vi "RPC Application.vi"() -> ()   [LabVIEW 2015]
uses:
  Classes/Request/Request.lvclass/Request.ctl
  Classes/Request/Read method.vi
  Classes/Request/Read params.vi
  <vilib>/NI/i3 JSON/JSON Generation/Create Value Files/Create Value - String.vi
  Classes/Server/Add Response (Method Not Found from Request).vi
  <vilib>/NI/i3 JSON/JSON Parsing/Get Array Value at Index Files/Get Array Value at Index - Numeric.vi
  <vilib>/NI/i3 JSON/JSON Generation/Create Value Files/Create Value - Numeric.vi
  Classes/Server/Add Response (Result from Request).vi
  Classes/Server/Add Response (Invalid Params from Request).vi
  Classes/Server/Add Response (Server Error from Request).vi
  Classes/params/params.lvclass
  Classes/Server/JSONRPC Server.lvclass
  <vilib>/NI/i3 JSON/i3-json.lvlib
  Classes/Request/Request.lvclass
panel:
  out "error out":errorcluster
  in  "error in (no error)":errorcluster
  # "To run this example:\n\nStart this VI\nRun \"RPC UI.vi\""
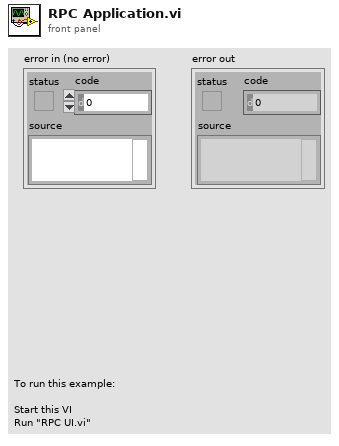
[diagram p1: front panel]
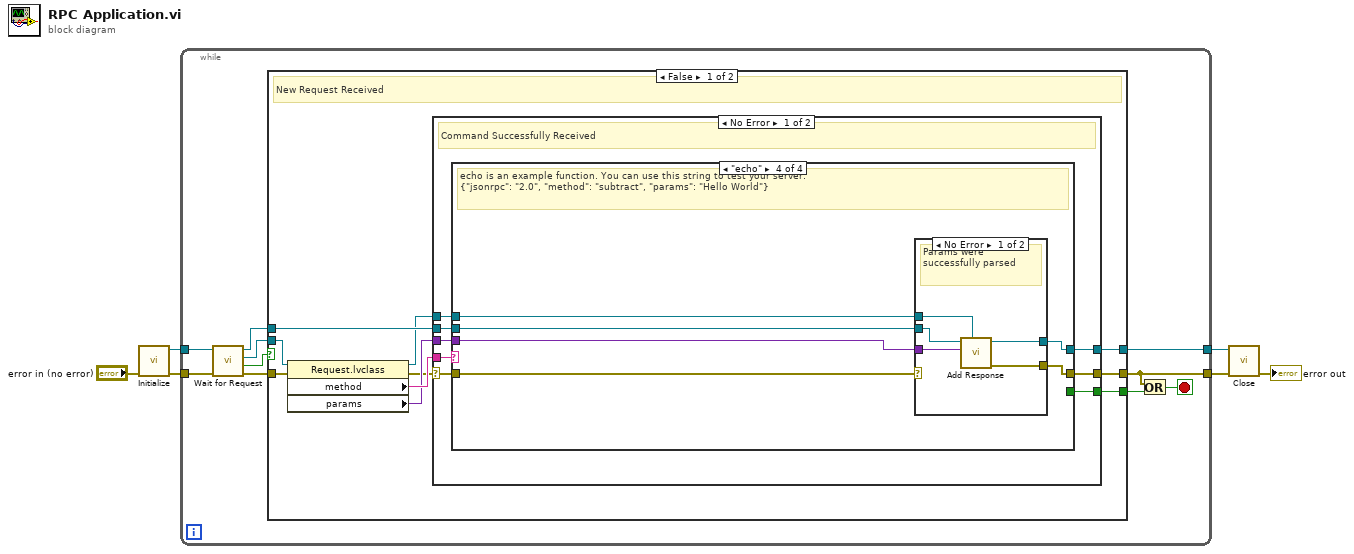
[diagram p0: block diagram]
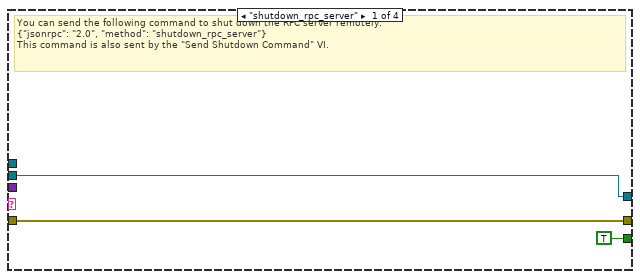
[diagram p2: hidden frame]
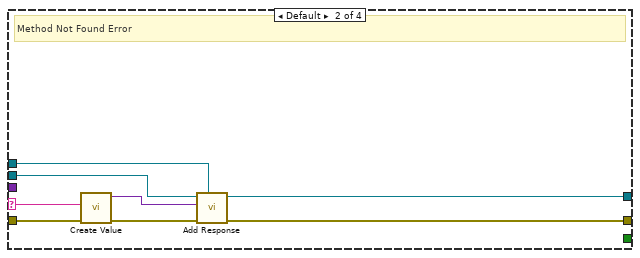
[diagram p3: hidden frame]
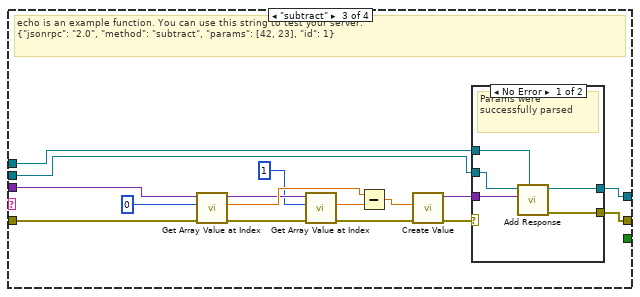
[diagram p4: hidden frame]
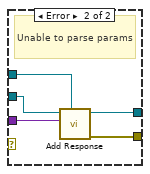
[diagram p5: hidden frame]
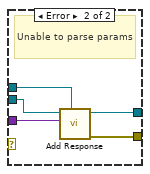
[diagram p6: hidden frame]
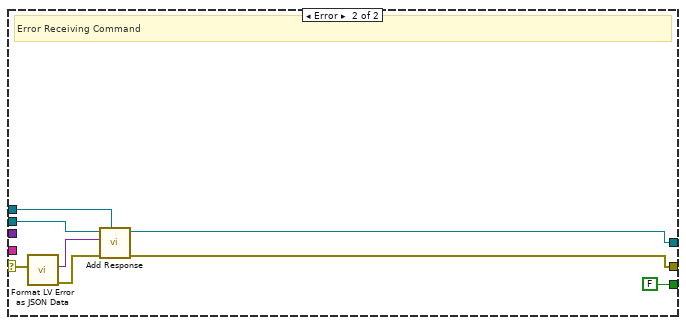
[diagram p7: hidden frame]
diagram:
  n1 = call "Initialize.vi"("error in (no error)"="error in (no error)") -> ("error out"=w2:errorcluster, "Server Out"=w1:refnum<class "JSONRPC Server.lvclass">)  [unwired: 9 in]
  n2 = while {
    tunnel: w1 -> [w16]
    tunnel: w2 -> [w12]
    tunnel: [w8] -> w4
    tunnel: [w10] -> w3
    stop <- w7 stop-if-true
    n3 = call "Wait for Request.vi"("error in (no error)"=w12, "Server in"=w16) -> ("error out"=w11:errorcluster, "timed out?"=w13:bool, "Request"=w14:refnum<class "Request.lvclass">, "Server out"=w15:refnum<class "JSONRPC Server.lvclass">)  [unwired: 6 in]
    n4 = case shown="False" w13 {
      tunnel: w15 -> [w19 w96]
      tunnel: w14 -> [w26 _]
      tunnel: w11 -> [w23 w97]
      tunnel: [w21 w97] -> w8
      tunnel: [w20 _] -> w9
      tunnel: [w18 w96] -> w10
      frame False {
        # "New Request Received"
        n5 = property class="Request.lvclass"(reference=w26, error in=w23) -> (reference out=w17:refnum<class "Request.lvclass">, error out=w22:errorcluster, "method"=w25:string, "params"=w24:variant)
        n6 = case shown="No Error" w22 {
          selector: w22 -> [w32 w89]
          tunnel: w25 -> [w34 _]
          tunnel: w24 -> [w33 _]
          tunnel: [w31 w92] -> w21
          tunnel: [w30 FALSE] -> w20
          tunnel: w19 -> [w29 w94]
          tunnel: [w28 w93] -> w18
          tunnel: w17 -> [w27 w95]
          frame No Error {
            # "Command Successfully Received"
            n7 = case shown="\"echo\"" w34 {
              selector: w34 -> [_ w43 _ _]
              tunnel: w33 -> [_ _ w58 w72]
              tunnel: w32 -> [w36 w39 w56 w73]
              tunnel: [w36 w41 w48 w75] -> w31
              tunnel: [TRUE _ _ _] -> w30
              tunnel: w29 -> [w35 w45 w51 w77]
              tunnel: [w35 w40 w50 w76] -> w28
              tunnel: w27 -> [_ w44 w47 w74]
              frame "shutdown_rpc_server" {
                # "You can send the following command to shut down the RPC server remotely:\n{\"jsonrpc\": \"2.0\", \"method\": \"shutdown_rpc_server\"}\nThis command is also sent by the \"Send Shutdown Command\" VI."
              }
              frame Default {
                # "Method Not Found Error"
                n8 = call-poly <vilib>:"Create Value.vi"("error in (no error)"=w39, "String"=w43) -> ("error out"=w38:errorcluster, "JSON Tree"=w42:variant)  [unwired: 8 in]
                n9 = call-poly "Add Response.vi"("Request"=w44, "error in (no error)"=w38, "data"=w42, "Server in"=w45) -> ("error out"=w41:errorcluster, "Server out"=w40:refnum<class "JSONRPC Server.lvclass">)  [unwired: 6 in]
              }
              frame "subtract" {
                # "echo is an example function. You can use this string to test your server:\n{\"jsonrpc\": \"2.0\", \"method\": \"subtract\", \"params\": [42, 23], \"id\": 1}"
                n10 = call-poly <vilib>:"Get Array Value at Index.vi"("error in (no error)"=w56, "Index"=0, "JSON Tree In (JSON Array)"=w58) -> ("error out"=w55:errorcluster, "Double Value"=w60:dbl, "JSON Tree Out Passthrough"=w57:variant)  [unwired: 5 in, 1 out]
                n11 = call-poly <vilib>:"Get Array Value at Index.vi"("error in (no error)"=w55, "Index"=1, "JSON Tree In (JSON Array)"=w57) -> ("error out"=w54:errorcluster, "Double Value"=w59:dbl)  [unwired: 5 in, 2 out]
                n12 = Subtract(x=w60, y=w59) -> (x-y=w61:dbl)
                n13 = call-poly <vilib>:"Create Value.vi"("error in (no error)"=w54, "Numeric"=w61) -> ("error out"=w46:errorcluster, "JSON Tree"=w49:variant)  [unwired: 8 in]
                n14 = case shown="No Error" w46 {
                  tunnel: w51 -> [w66 w71]
                  tunnel: [w65 w70] -> w50
                  tunnel: w49 -> [w64 w69]
                  tunnel: [w63 w68] -> w48
                  tunnel: w47 -> [w62 w67]
                  frame No Error {
                    # "Params were successfully parsed"
                    n15 = call-poly "Add Response.vi"("Request"=w62, "Response JSON Tree In"=w64, "Server in"=w66) -> ("error out"=w63:errorcluster, "Server out"=w65:refnum<class "JSONRPC Server.lvclass">)  [unwired: 7 in]
                  }
                  frame Error {
                    # "Unable to parse params"
                    n16 = call-poly "Add Response.vi"("Request"=w67, "data"=w69, "Server in"=w71) -> ("error out"=w68:errorcluster, "Server out"=w70:refnum<class "JSONRPC Server.lvclass">)  [unwired: 7 in]
                  }
                }
              }
              frame "echo" {
                # "echo is an example function. You can use this string to test your server:\n{\"jsonrpc\": \"2.0\", \"method\": \"subtract\", \"params\": \"Hello World\"}"
                n17 = case shown="No Error" w73 {
                  tunnel: w77 -> [w82 w87]
                  tunnel: [w81 w86] -> w76
                  tunnel: w72 -> [w80 w85]
                  tunnel: [w79 w84] -> w75
                  tunnel: w74 -> [w78 w83]
                  frame No Error {
                    # "Params were successfully parsed"
                    n18 = call-poly "Add Response.vi"("Request"=w78, "Response JSON Tree In"=w80, "Server in"=w82) -> ("error out"=w79:errorcluster, "Server out"=w81:refnum<class "JSONRPC Server.lvclass">)  [unwired: 7 in]
                  }
                  frame Error {
                    # "Unable to parse params"
                    n19 = call-poly "Add Response.vi"("Request"=w83, "data"=w85, "Server in"=w87) -> ("error out"=w84:errorcluster, "Server out"=w86:refnum<class "JSONRPC Server.lvclass">)  [unwired: 7 in]
                  }
                }
              }
            }
          }
          frame Error {
            # "Error Receiving Command"
            n20 = call "Format LV Error as JSON Data.vi"("error in"=w89) -> ("error out"=w90:errorcluster, "Error Data Out"=w88:variant)  [unwired: 9 in]
            n21 = call-poly "Add Response.vi"("Request"=w95, "error in (no error)"=w90, "data"=w88, "Server in"=w94) -> ("error out"=w92:errorcluster, "Server out"=w93:refnum<class "JSONRPC Server.lvclass">)  [unwired: 6 in]
          }
        }
      }
      frame True {
        # "Timeout while waiting for new Requests"
      }
    }
    n22 = Or(x=w8, y=w9) -> (x .or. y?=w7:bool)
  }
  n23 = call-dynamic "Close.vi"("error in (no error)"=w4, "Server in"=w3) -> ("error out"=→"error out":errorcluster)  [unwired: 9 in]
